vi "TEST angle adjustments for front and field.vi"() -> ()   [LabVIEW 2023]
uses:
  ctrl defs/ctrl DRIVING FRAME selector.ctl
  ctrl defs/ctrl FRONT FACE selector.ctl
  <vilib>/Rock Robotics/WPI/DriverStation/WPI_DriverStationAllianceInfo.ctl
  Global odometry.vi
panel:
  out "MAGNETIC Zero for Blue Alliance (deg)":dbl=200.5 format="%#.4f"
  out "front facing\noffset":dbl
  in  "Alliance":T1
  in  "front\nface":T2
  out "drive angle (deg)\nwrt +X on robot":dbl(knob)
  in  "drive frame":T3
  in  "Joystick angle (deg CCW)":dbl(slide)
  in  "stop":bool
  in  "ROBOT compass reading (deg CW)":dbl(slide)
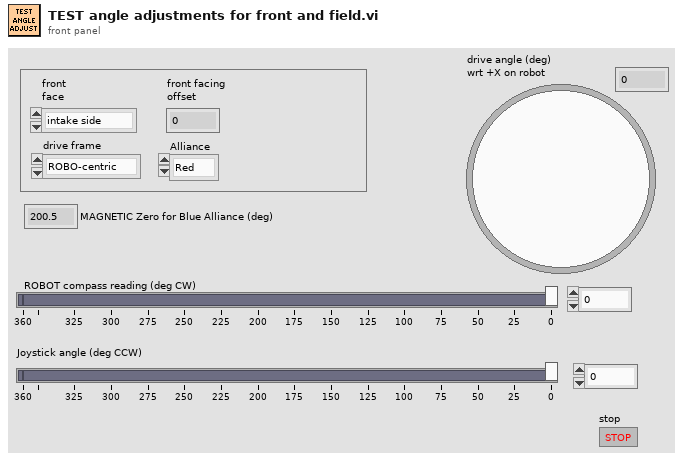
[diagram p1: front panel]
types:
  T1 = typedef "WPI_DriverStationAllianceInfo.ctl" = enum16{"Red", "Blue", "Invalid"}
  T2 = typedef "ctrl FRONT FACE selector.ctl" = enum16{"intake side", "shooter side"}
  T3 = typedef "ctrl DRIVING FRAME selector.ctl" = enum16{"ROBO-centric", "FLD-centric"}
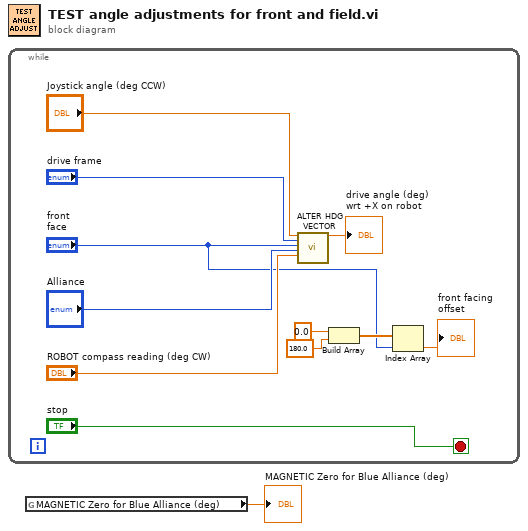
[diagram p0: block diagram]
diagram:
  n1 = while {
    stop <- "stop" stop-if-true
    n2 = call "ALTER HDG VECTOR.vi"("Joystick angle (deg CCW)"="Joystick angle (deg CCW)", "drive frame"="drive frame", "front face"="front\nface", "Alliance"="Alliance", "ROBOT compass reading (deg CW)"="ROBOT compass reading (deg CW)") -> ("Joystick (deg)"=→"drive angle (deg)\nwrt +X on robot":dbl)  [unwired: 14 in]
    n3 = Build Array(0.0 ("element"), 180.0 ("element")) -> (w4:dbl[])
    n4 = Index Array(array=w4, index="front\nface") -> (element=→"front facing\noffset":dbl)
  }
  n5 = global read "Global odometry.vi" "MAGNETIC Zero for Blue Alliance (deg)"() -> (→"MAGNETIC Zero for Blue Alliance (deg)":dbl)
